vi "number3-insertion sort.vi"(3 "Boolean":bool=TRUE, 4 "Array":dbl[](array[numeric]), 5 "Wait":u32=10) -> (1 "Waveform Graph":dbl[](graph))   [LabVIEW 2014]
panel:
  in  "Number of Elements":i32=1024
  out "element":dbl
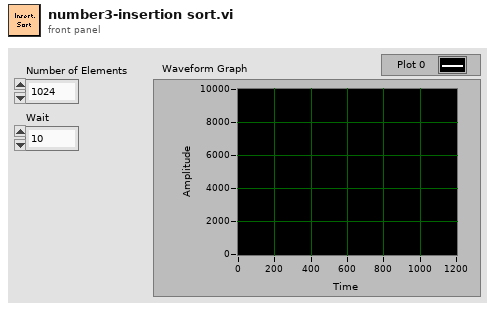
[diagram p1: front panel]
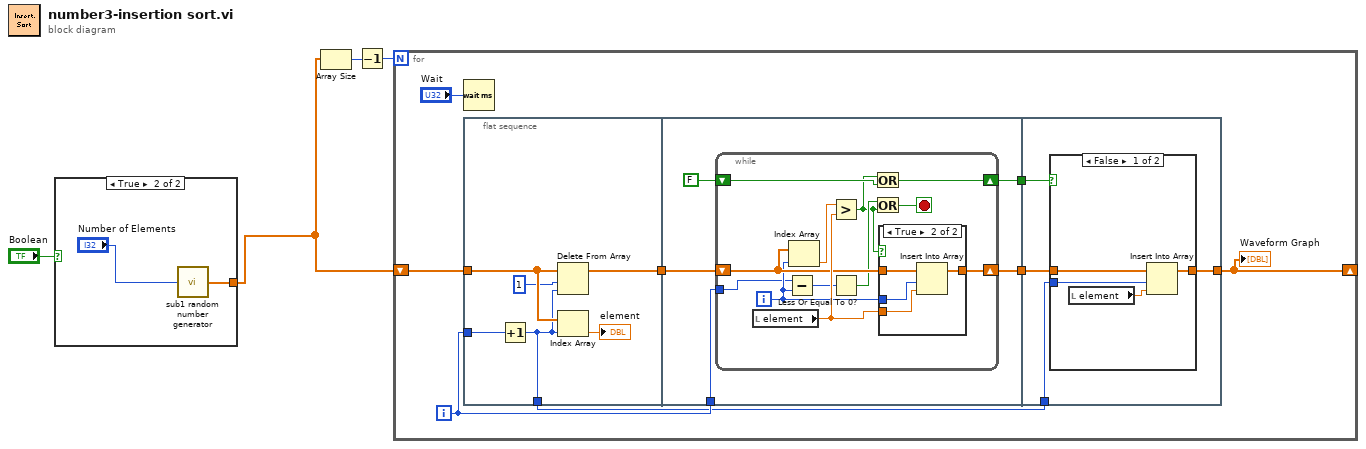
[diagram p0: block diagram]
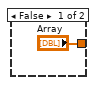
[diagram p2: hidden frame]
diagram:
  n1 = case shown="True" "Boolean" {
    tunnel: ["Array" w7] -> w1
    frame False {
    }
    frame True {
      n2 = call "sub1 random number generator.vi"("Numeric"="Number of Elements") -> ("Array"=w7:dbl[])  [unwired: 4 in]
    }
  }
  n3 = Array Size(array=w1) -> (size(s)=w4:i32)
  n4 = Decrement(x=w4) -> (x-1=w3:i32)
  n5 = for {
    N: w3 -> [_]
    shift-right: [w10] -> _
    shift-left: w1 -> [w15]
    i -> [w11]
    n6 = Wait (ms)(milliseconds to wait="Wait") -> ()  [unwired: 1 out]
    n7 = flat-sequence {
      tunnel: w11 -> [w21]
      tunnel: w15 -> [w19]
      tunnel: [w17] -> w14
      tunnel: [w16] -> w9
      tunnel: w14 -> [w26]
      tunnel: [w25] -> w13
      tunnel: [w23] -> w12
      tunnel: w11 -> [w22]
      tunnel: w13 -> [w46]
      tunnel: w12 -> [w47]
      tunnel: [w45] -> w10
      tunnel: w9 -> [w44]
      frame #0 {
        n8 = Increment(x=w21) -> (x+1=w16:i32)
        n9 = Delete From Array(array=w19, length=1, index=w16) -> (array with subset deleted=w17:dbl[])  [unwired: 1 out]
        n10 = Index Array(array=w19, index=w16) -> (element=→"element":dbl)
      }
      frame #1 {
        n11 = while {
          shift-right: [w37] -> w25
          shift-left: w26 -> [w35]
          shift-right: [w33] -> w23
          shift-left: FALSE -> [w31]
          tunnel: w22 -> [w28]
          i -> [w29]
          stop <- w34 stop-if-true
          n12 = local read "element"() -> (w36:dbl)
          n13 = Subtract(x=w28, y=w29) -> (x-y=w27:i32)
          n14 = Index Array(array=w35, index=w29) -> (element=w38:dbl)
          n15 = Greater?(x=w38, y=w36) -> (0:w30:bool)
          n16 = Less Or Equal To 0?(x=w27) -> (x <= 0?=w32:bool)
          n17 = Or(x=w30, y=w31) -> (x .or. y?=w33:bool)
          n18 = Or(x=w32, y=w30) -> (x .or. y?=w34:bool)
          n19 = case shown="True" w30 {
            tunnel: w35 -> [w39 w43]
            tunnel: [w39 w42] -> w37
            tunnel: w29 -> [_ w41]
            tunnel: w36 -> [_ w40]
            frame False {
            }
            frame True {
              n20 = Insert Into Array(array=w43, index=w41, new element=w40) -> (w42:dbl[])
            }
          }
        }
      }
      frame #2 {
        n21 = case shown="False" w47 {
          tunnel: w46 -> [w51 w52]
          tunnel: [w49 w52] -> w45
          tunnel: w44 -> [w48 _]
          frame False {
            n22 = local read "element"() -> (w50:dbl)
            n23 = Insert Into Array(array=w51, index=w48, new element=w50) -> (w49:dbl[])
          }
          frame True {
          }
        }
      }
    }
    "Waveform Graph" <- w10
  }
